vi "H5PTget_next.vi"(5 "data":i32[](array[numeric]), 7 "nrecords":i64, 8 "error in (no error)":errorcluster, 11 "table_id":i32) -> (0 "error out":errorcluster, 3 "status":i32)   [LabVIEW 2009]
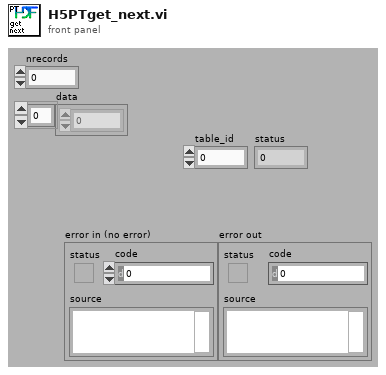
[diagram p1: front panel]
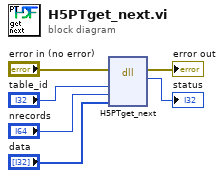
[diagram p0: block diagram]
diagram:
  n1 = dll-call lib="hdf5_hldll" fn="H5PTget_next"(error in="error in (no error)", "table_id"="table_id", "nrecords"="nrecords", "data"="data") -> (error out=→"error out":errorcluster, "return type"=→"status":i32)  [unwired: 5 in, 1 out]
